vi "SetRandomPoint.vi"(8 "error in (no error)":errorcluster, 11 "Snake in":refnum<class "SnakeGame.lvclass">) -> (0 "error out":errorcluster, 3 "Snake out":refnum<class "SnakeGame.lvclass">)   [LabVIEW 2019]
uses:
  SnakeGame.lvclass
  C:/Users/FreshBob/Dropbox/VIs/myRIO_GameConsole/RT/RT_Game/Game/Game.lvclass
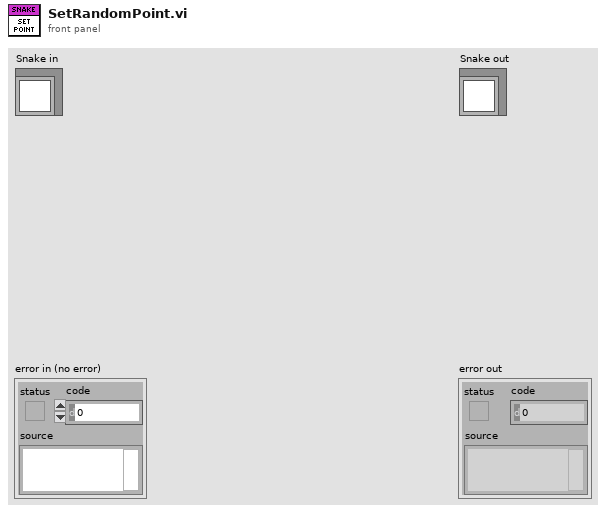
[diagram p1: front panel]
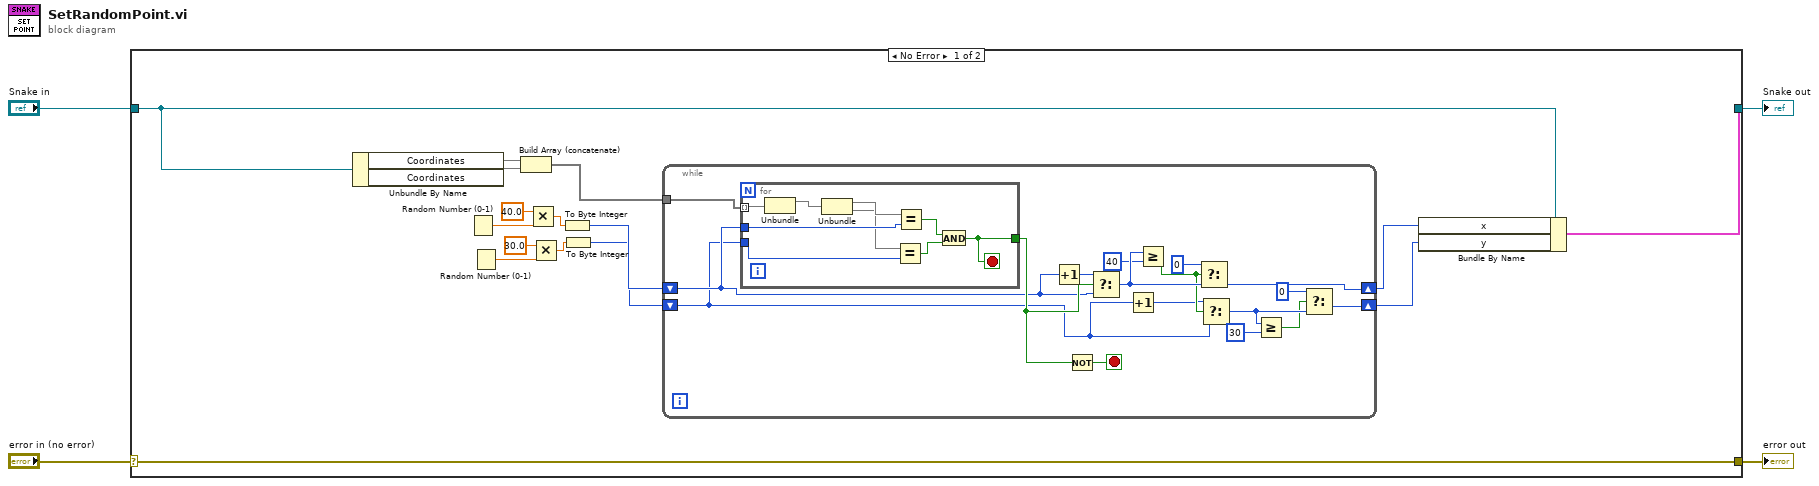
[diagram p0: block diagram]
diagram:
  n1 = case shown="No Error" "error in (no error)" {
    selector: "error in (no error)" -> [w20 w48]
    tunnel: [w20 w48] -> w3
    tunnel: [w19 w47] -> w1
    tunnel: "Snake in" -> [w12 w47]
    frame No Error {
      n2 = Unbundle By Name(w12) -> ("Coordinates"=w9, "Coordinates"=w5)
      n3 = Random Number (0-1)() -> (number: 0 to 1=w18:dbl)
      n4 = Random Number (0-1)() -> (number: 0 to 1=w14:dbl)
      n5 = Build Array (concatenate)(w9, w5) -> (w6:void[])
      n6 = Multiply(x=40.0, y=w18) -> (x*y=w16:dbl)
      n7 = Multiply(x=30.0, y=w14) -> (x*y=w13:dbl)
      n8 = To Byte Integer(number=w16) -> (8bit integer=w11:i8)
      n9 = To Byte Integer(number=w13) -> (8bit integer=w10:i8)
      n10 = while {
        shift-right: [w30] -> w8
        shift-left: w11 -> [w34]
        shift-right: [w23] -> w7
        shift-left: w10 -> [w27]
        tunnel: w6 -> [w37]
        stop <- w35 stop-if-true
        n11 = for {
          tunnel: w37 -> [w46] mode=indexing
          tunnel: w34 -> [w45]
          tunnel: w27 -> [w44]
          tunnel: [w41] -> w36
          stop <- w41 stop-if-true
          n12 = Unbundle(w46) -> (w40)  [unwired: 1 out]
          n13 = Unbundle(w40) -> (w39, w38)
          n14 = Equal?(x=w38, y=w44) -> (x = y?=w43:bool)
          n15 = Equal?(x=w39, y=w45) -> (x = y?=w42:bool)
          n16 = And(x=w42, y=w43) -> (x .and. y?=w41:bool)
        }
        n17 = Increment(x=w34) -> (x+1=w33:i8)
        n18 = Not(x=w36) -> (.not. x?=w35:bool)
        n19 = Select(t=w33, s=w36, f=w34) -> (s? t:f=w32:i8)
        n20 = Increment(x=w27) -> (x+1=w26:i8)
        n21 = Greater Or Equal?(x=w32, y=i8 40 ("x")) -> (x >= y?=w28:bool)
        n22 = Select(t=i8 0, s=w28, f=w32) -> (s? t:f=w30:i8)
        n23 = Select(t=w26, s=w28, f=w27) -> (s? t:f=w25:i8)
        n24 = Greater Or Equal?(x=w25, y=i8 30) -> (x >= y?=w22:bool)
        n25 = Select(t=i8 0, s=w22, f=w25) -> (s? t:f=w23:i8)
      }
      n26 = Bundle By Name(cluster=w12, "x"=w8, "y"=w7) -> (w19:cluster{})
    }
    frame Error {
    }
  }
  "error out" <- w3
  "Snake out" <- w1
